vi "Set Channels Config Analog In.vi"(5 "voltOffset":dbl, 6 "Filter":T1, 7 "voltsRange":dbl, 8 "error in (no error)":errorcluster, 9 "Enable":i32, 10 "indexCh":i32, 11 "hdwf":i32) -> (0 "error out":errorcluster, 1 "function return":i32, 3 "hdwf out":i32)   [LabVIEW 2012, in "AnalogDiscSDKLv.lvlib"]
doc: "extern \"C\" __declspec(dllexport) int SetChannelsConfig_AnalogIn(HDWF hdwf, \n int indexCh, int Enable, double voltsRange, FILTER Filter, double voltOffset );"
uses:
  <instrlib>/AnalogDiscSDKLv/AnalogDiscSDKLv.lvlib
  <instrlib>/AnalogDiscSDKLv/VIs/DWF_Filter.ctl
  <instrlib>/AnalogDiscSDKLv/AnalogDiscSDKLv.dll
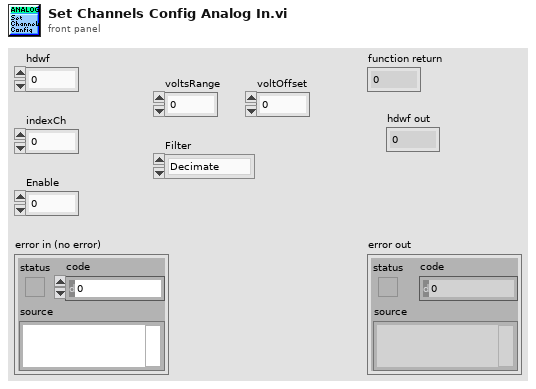
[diagram p1: front panel]
types:
  T1 = typedef "DWF_Filter.ctl" = enum16{"Decimate", "Average", "MinMax"}
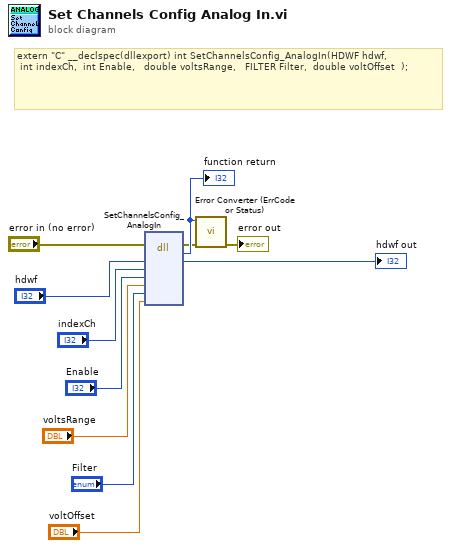
[diagram p0: block diagram]
diagram:
  # "extern \"C\" __declspec(dllexport) int SetChannelsConfig_AnalogIn(HDWF hdwf, \n\tint indexCh,\t\tint Enable,\t\t\tdouble voltsRange,\t\t\tFILTER Filter,\t\tdouble voltOffset\t\t);"
  n1 = dll-call lib="C:/Program Files (x86)/National Instruments/LabVIEW 2012/instr.lib/AnalogDiscSDKLv/AnalogDiscSDKLv.*" fn="SetChannelsConfig_AnalogIn"(error in="error in (no error)", "hdwf"="hdwf", "indexCh"="indexCh", "Enable"="Enable", "voltsRange"="voltsRange", "Filter"="Filter", "voltOffset"="voltOffset") -> (error out=w4:errorcluster, w11:i32, "hdwf"=→"hdwf out":i32)  [unwired: 7 in, 1 out]
  "function return" <- w11
  n2 = call <instrlib>:"Error Converter (ErrCode or Status).vi"("error in (no error)"=w4, "error code"=w11) -> ("error out"=→"error out":errorcluster)  [unwired: 9 in]
